vi "_Obtain JKISMQ.vi"(8 "Error in":errorcluster caption="Error in (no error)", 9 "create if not found? (T)":bool=TRUE, 11 "Name(\"\" to use uuid) in":string) -> (0 "Error out":errorcluster, 1 "Stand Alone Mode":bool, 3 "JKISMQ":T1, 4 "Name":string)   [LabVIEW 2020, in "JKI-State-Machine-Plus.lvlib"]
uses:
  JKI-State-Machine-Plus.lvlib
  _JKISMQ.ctl
  _Cross JKI StateMachine State Data.ctl
  _Cross JKI StateMachine State Response.ctl
  _JKISMQFGVOPER.ctl
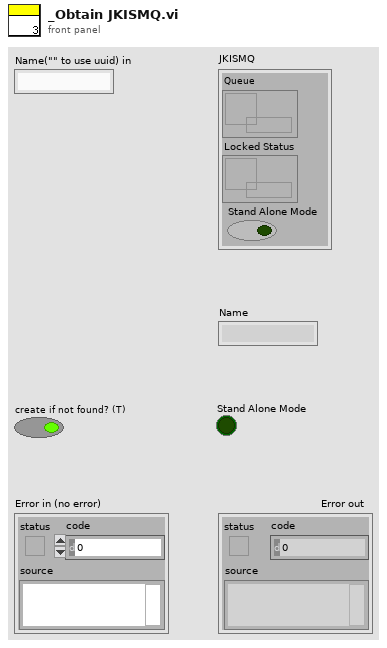
[diagram p1: front panel]
types:
  T1 = typedef "JKI-State-Machine-Plus.lvlib/_JKISMQ.ctl" = cluster{"Queue":refnum<queue>, "Locked Status":refnum<data-value>, "Stand Alone Mode":bool}
  T2 = typedef "JKI-State-Machine-Plus.lvlib/_JKISMQFGVOPER.ctl" = enum16{"Get By Name", "List"}
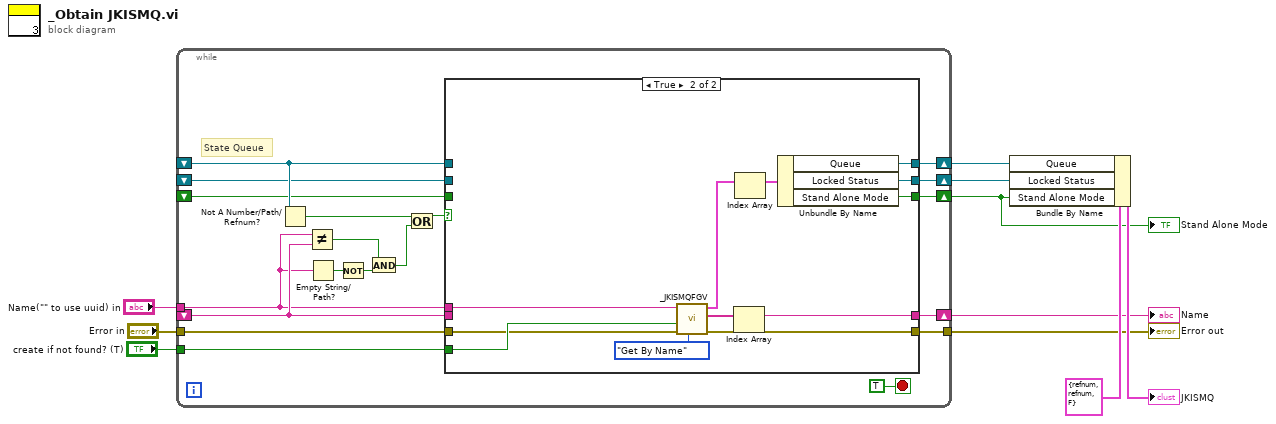
[diagram p0: block diagram]
diagram:
  n1 = while {
    shift-right: [w28] -> w6
    shift-left: _ -> [w26]
    shift-right: [w25] -> w5
    shift-left: _ -> [w17]
    shift-right: [w24] -> w8
    shift-left: _ -> [w23]
    shift-right: [w22] -> w7
    shift-left: _ -> [w21]
    tunnel: "create if not found? (T)" -> [w20]
    tunnel: "Error in" -> [w19]
    tunnel: [w18] -> w2
    tunnel: "Name(\"\" to use uuid) in" -> [w12]
    stop <- TRUE stop-if-true
    # "State Queue"
    n2 = Not A Number/Path/Refnum?(number/path/refnum=w26) -> (NaN/Path/Refnum?=w27:bool)
    n3 = Not Equal?(x=w12, y=w17) -> (x != y?=w15:bool)
    n4 = Empty String/Path?(string/path=w12) -> (empty?=w13:bool)
    n5 = Not(x=w13) -> (.not. x?=w11:bool)
    n6 = And(x=w15, y=w11) -> (x .and. y?=w14:bool)
    n7 = Or(x=w27, y=w14) -> (x .or. y?=w16:bool)
    n8 = case shown="True" w16 {
      tunnel: w17 -> [w33 _]
      tunnel: [w34 w44] -> w28
      tunnel: w26 -> [w34 _]
      tunnel: [w33 w36] -> w25
      tunnel: [w32 w43] -> w24
      tunnel: w23 -> [w32 _]
      tunnel: [w31 w45] -> w22
      tunnel: w21 -> [w31 _]
      tunnel: w20 -> [_ w42]
      tunnel: w19 -> [w30 w39]
      tunnel: [w30 w38] -> w18
      tunnel: w12 -> [_ w35]
      frame False {
      }
      frame True {
        n9 = call "_JKISMQFGV.vi"("Enum"=_JKISMQFGVOPER."Get By Name", "Error in"=w39, "create if not found? (T)"=w42, "Name(\"\" to use uuid) in"=w35) -> ("Error out"=w38:errorcluster, "Name"=w40:string[], "Array"=w46:T1[])  [unwired: 5 in]
        n10 = Index Array(array=w40) -> (element=w36:string)  [unwired: 1 in]
        n11 = Index Array(array=w46) -> (element=w37:T1)  [unwired: 1 in]
        n12 = Unbundle By Name(w37) -> ("Queue"=w44:refnum<queue>, "Locked Status"=w45:refnum<data-value>, "Stand Alone Mode"=w43:bool)
      }
    }
  }
  "Error out" <- w2
  "Name" <- w5
  "Stand Alone Mode" <- w8
  n13 = Bundle By Name(cluster=T1 {"Queue"=refnum, "Locked Status"=refnum, "Stand Alone Mode"=FALSE} ("JKISMQ"), "Queue"=w6, "Locked Status"=w7, "Stand Alone Mode"=w8) -> (→"JKISMQ":T1)
